vi "Make ramps.vi"(0 "Final positions (deg)":dbl[](array[numeric])=[5.0, 10.0, 20.0], 2 "Ramp velocities (deg/s)":dbl[](array[numeric])=[5.0, 10.0], 3 "Direction":dbl[](array[numeric])=[1.0, -1.0], 5 "Hold time (s)":dbl[](array[numeric]), 8 "Repetitions":i32=2, 9 "randomize":bool=TRUE, 10 "gap time (s)":dbl, 11 "sampling rate":dbl) -> (14 "sine signal":dbl[](array[numeric]), 15 "ramp data":T1, 16 "ramp signal":dbl[](array[numeric]), 17 "stimphases":T2, 19 "Total time":dbl)   [LabVIEW 2013]
uses:
  Phases.ctl
  Pulse data.ctl
  <vilib>/Analysis/1siggen.llb/Ramp Pattern by Samples.vi
  <vilib>/Analysis/NI_AALBase.lvlib
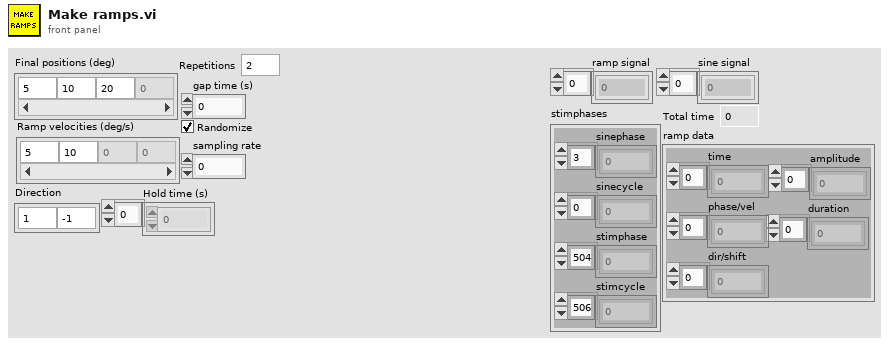
[diagram p1: front panel]
types:
  T1 = typedef "Pulse data.ctl" = cluster{"time":dbl[], "phase/vel":dbl[], "dir/shift":dbl[], "amplitude":dbl[], "duration":dbl[]}
  T2 = typedef "Phases.ctl" = cluster{"sinephase":dbl[], "sinecycle":dbl[], "stimphase":dbl[], "stimcycle":dbl[]}
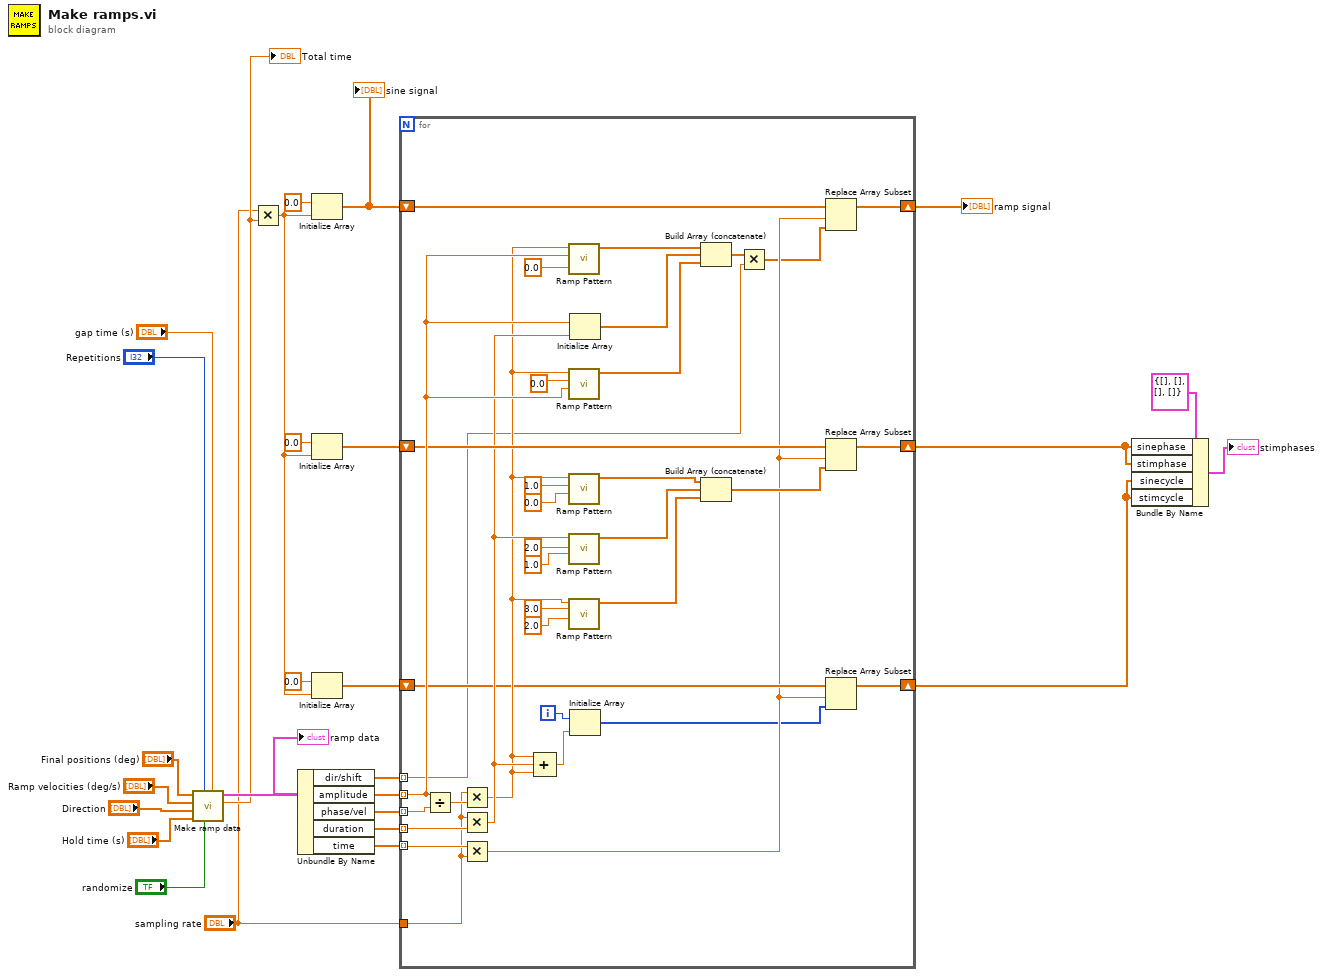
[diagram p0: block diagram]
diagram:
  n1 = call "Make ramp data.vi"("gap time (s)"="gap time (s)", "randomize"="randomize", "Repetitions"="Repetitions", "Hold time (s)"="Hold time (s)", "Directions"="Direction", "Ramp velocities (deg/s)"="Ramp velocities (deg/s)", "Final positions (deg)"="Final positions (deg)") -> ("Total time"=w19:dbl, "ramp data"=w20:T1)  [unwired: 3 in]
  "Total time" <- w19
  "ramp data" <- w20
  n2 = Multiply(x="sampling rate", y=w19) -> (x*y=w7:dbl)
  n3 = Unbundle By Name(w20) -> ("dir/shift"=w1:dbl[], "amplitude"=w17:dbl[], "phase/vel"=w16:dbl[], "duration"=w15:dbl[], "time"=w14:dbl[])
  n4 = Initialize Array(0.0 ("element"), w7) -> (w13:dbl[])
  "sine signal" <- w13
  n5 = Initialize Array(0.0 ("element"), w7) -> (w9:dbl[])
  n6 = Initialize Array(0.0 ("element"), w7) -> (w6:dbl[])
  n7 = for {
    tunnel: w17 -> [w58] mode=indexing
    tunnel: "sampling rate" -> [w53]
    tunnel: w16 -> [w63] mode=indexing
    tunnel: w15 -> [w60] mode=indexing
    tunnel: w14 -> [w54] mode=indexing
    shift-right: [w50] -> w12
    shift-left: w13 -> [w52]
    shift-right: [w38] -> w3
    shift-left: w9 -> [w42]
    shift-right: [w33] -> w2
    shift-left: w6 -> [w32]
    tunnel: w1 -> [w28] mode=indexing
    i -> [w37]
    n8 = Divide(x=w58, y=w63) -> (x/y=w62:dbl)
    n9 = Multiply(x=w53, y=w62) -> (x*y=w34:dbl)
    n10 = Multiply(x=w53, y=w60) -> (x*y=w35:dbl)
    n11 = Multiply(x=w54, y=w53) -> (x*y=w31:dbl)
    n12 = Compound Arithmetic op=ADD(w34, w35, w34) -> (w36:dbl)
    n13 = call-poly <vilib>:"Ramp Pattern.vi"("start"=0.0, "end"=w58, "samples"=w34) -> ("Ramp Pattern"=w57:dbl[])  [unwired: 7 in, 1 out]
    n14 = call-poly <vilib>:"Ramp Pattern.vi"("start"=w58, "end"=0.0 ("start"), "samples"=w34) -> ("Ramp Pattern"=w55:dbl[])  [unwired: 7 in, 1 out]
    n15 = call-poly <vilib>:"Ramp Pattern.vi"("start"=0.0, "end"=1.0 ("start"), "samples"=w34) -> ("Ramp Pattern"=w41:dbl[])  [unwired: 7 in, 1 out]
    n16 = call-poly <vilib>:"Ramp Pattern.vi"("start"=1.0, "end"=2.0 ("start"), "samples"=w35) -> ("Ramp Pattern"=w40:dbl[])  [unwired: 7 in, 1 out]
    n17 = call-poly <vilib>:"Ramp Pattern.vi"("start"=2.0, "end"=3.0 ("start"), "samples"=w34) -> ("Ramp Pattern"=w39:dbl[])  [unwired: 7 in, 1 out]
    n18 = Initialize Array(w58, w35) -> (w56:dbl[])
    n19 = Initialize Array(w37, w36) -> (w30:i32[])
    n20 = Build Array (concatenate)(w57, w56, w55) -> (w51:dbl[])
    n21 = Build Array (concatenate)(w41, w40, w39) -> (w43:dbl[])
    n22 = Multiply(x=w51, y=w28) -> (x*y=w29:dbl[])
    n23 = Replace Array Subset(array=w52, new element=w29, index=w31) -> (w50:dbl[])
    n24 = Replace Array Subset(array=w42, new element=w43, index=w31) -> (w38:dbl[])
    n25 = Replace Array Subset(array=w32, new element=w30, index=w31) -> (w33:dbl[])
  }
  "ramp signal" <- w12
  n26 = Bundle By Name(cluster=T2 {"sinephase"=[], "sinecycle"=[], "stimphase"=[], "stimcycle"=[]} ("stimphases"), "sinephase"=w3, "stimphase"=w3, "sinecycle"=w2, "stimcycle"=w2) -> (→"stimphases":T2)
